vi "Correlation_Setup.vi"(0 "Input string":string) -> (1 "Correlate":i32[][](array[numeric]), 2 "Error?":bool)   [LabVIEW 2010]
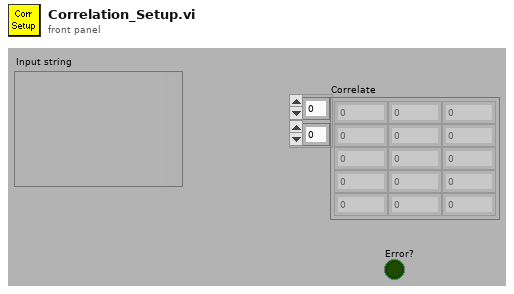
[diagram p1: front panel]
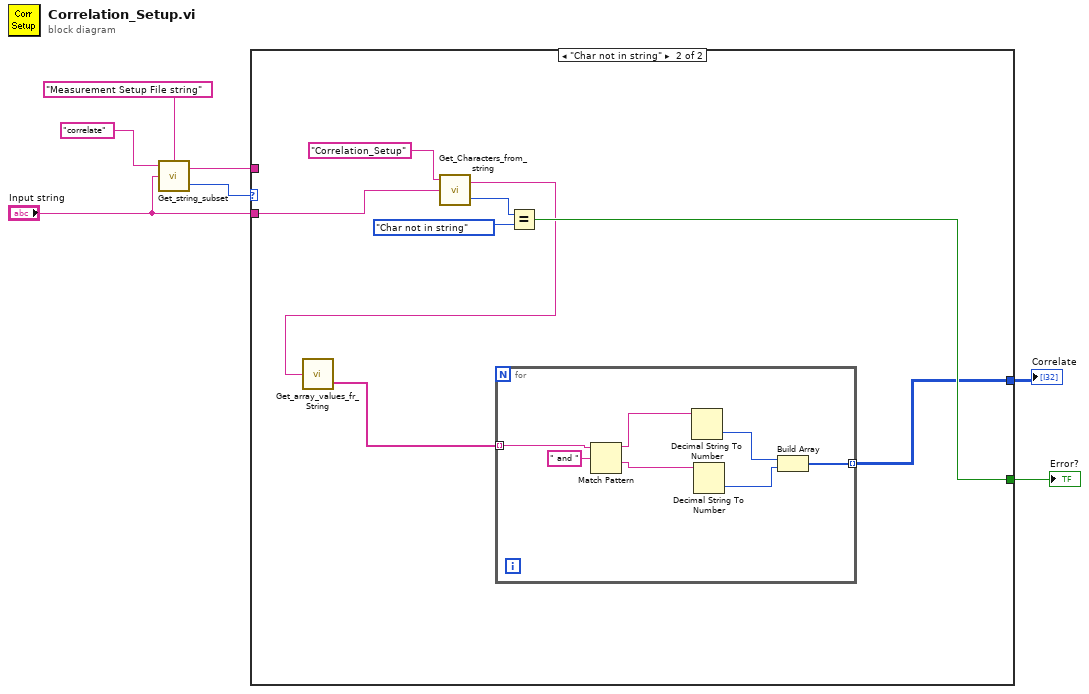
[diagram p0: block diagram]
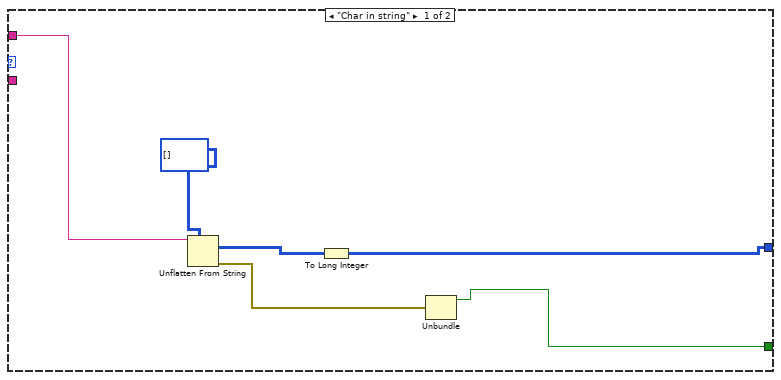
[diagram p2: hidden frame]
diagram:
  n1 = call "Get_string_subset.vi"("String Name"="Measurement Setup File string", "String to split"="Input string", "File Label"="correlate") -> ("Status"=w5:enum16{"Char in string", "Char not in string"}, "Output string"=w4:string)  [unwired: 1 in]
  n2 = case shown="\"Char not in string\"" w5 {
    tunnel: "Input string" -> [_ w21]
    tunnel: w4 -> [w8 _]
    tunnel: [w9 w14] -> w2
    tunnel: [w10 w17] -> w3
    frame "Char in string" {
      n3 = Unflatten From String(type=i8[][] [] ("correlate"), binary string=w8) -> (value=w12:i8[][], error out=w11:errorcluster)  [unwired: 1 in, 3 out]
      n4 = To Long Integer(number=w12) -> (32bit integer=w9:i32[][])
      n5 = Unbundle(w11) -> ("status"=w10:bool)  [unwired: 2 out]
    }
    frame "Char not in string" {
      n6 = call "Get_Characters_from_string.vi"("Input string"=w21, "Variable name"="Correlation_Setup") -> ("Status"=w18:enum16{"Char in string", "Char not in string"}, "Value"=w16:string)  [unwired: 1 in]
      n7 = call "Get_array_values_fr_String.vi"("String Value"=w16) -> ("String array"=w15:string[])  [unwired: 1 out]
      n8 = for {
        tunnel: w15 -> [w27] mode=indexing
        tunnel: [w22] -> w14 mode=indexing
        n9 = Match Pattern(string=w27, regular expression=" and ") -> (before substring=w26:string, after substring=w25:string)  [unwired: 3 out]
        n10 = Decimal String To Number(string=w26) -> (number=w24:i32)  [unwired: 3 out]
        n11 = Decimal String To Number(string=w25) -> (number=w23:i32)  [unwired: 3 out]
        n12 = Build Array(w24, w23) -> (w22:i32[])
      }
      n13 = Equal?(x=w18, y=enum16{"Char in string", "Char not in string"}."Char not in string" ("Status")) -> (x = y?=w17:bool)
    }
  }
  "Correlate" <- w2
  "Error?" <- w3
